vi "res_STRING_offset.vi"(7 "Serialized by PLC? (F)":bool, 10 "ST_results_info":T1, 11 "STRING_position":i32) -> (3 "results_byte_array_offset":i32)   [LabVIEW 2020]
uses:
  ST_results_info.ctl
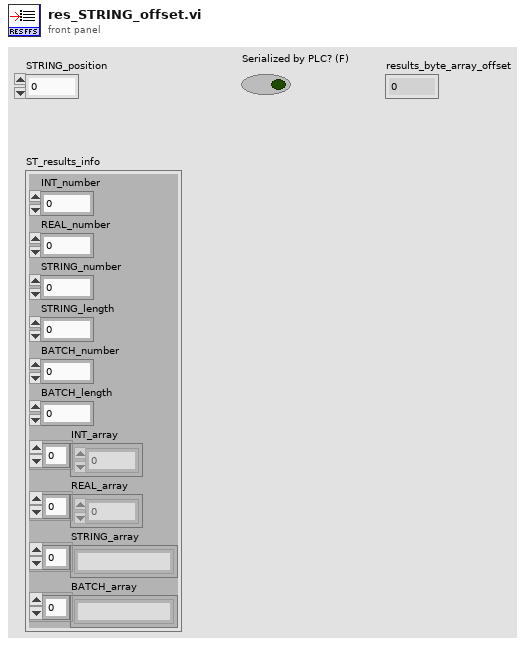
[diagram p1: front panel]
types:
  T1 = typedef "ST_results_info.ctl" = cluster{"INT_number":i32, "REAL_number":i32, "STRING_number":i32, "STRING_length":i32, "BATCH_number":i32, "BATCH_length":i32, "INT_array":i16[], "REAL_array":sgl[], "STRING_array":string[], "BATCH_array":string[]}
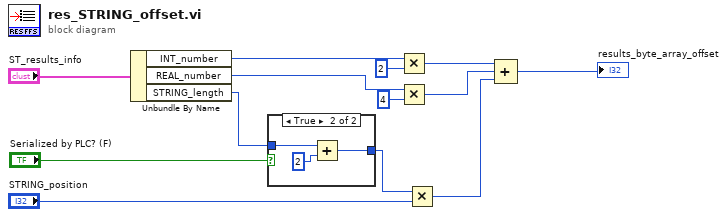
[diagram p0: block diagram]
diagram:
  n1 = Unbundle By Name("ST_results_info") -> ("INT_number"=w12:i32, "REAL_number"=w10:i32, "STRING_length"=w4:i32)
  n2 = case shown="True" "Serialized by PLC? (F)" {
    tunnel: w4 -> [w14 w17]
    tunnel: [w14 w15] -> w2
    frame False {
    }
    frame True {
      n3 = Add(x=w17, y=2) -> (x+y=w15:i32)
    }
  }
  n4 = Multiply(x=w12, y=2) -> (x*y=w8:i32)
  n5 = Multiply(x=w10, y=4) -> (x*y=w7:i32)
  n6 = Multiply(x=w2, y="STRING_position") -> (x*y=w6:i32)
  n7 = Compound Arithmetic op=ADD(w8, w7, w6) -> (→"results_byte_array_offset":i32)
